vi "Add Points to Series_DBL-DBL[].vi"(6 "YValuesPerPoint":i32=1, 8 "error in (no error)":errorcluster, 9 "Data":cluster{"X":dbl, "Y":dbl[]}[](array[cluster])=[{"X"=0.0, "Y"=[]}, {"X"=0.0, "Y"=[]}, {"X"=0.0, "Y"=[]}, {"X"=0.0, "Y"=[]}, {"X"=0.0, "Y"=[]}, {"X"=0.0, "Y"=[]}, {"X"=0.0, "Y"=[]}, {"X"=0.0, "Y"=[]}], 10 ".NET MSChart Series":refnum<k24>) -> (0 "error out":errorcluster, 2 ".NET MSChart Series (dup)":refnum<k24>)   [LabVIEW 2014, in "XMSChart.xctl"]
uses:
  XMSChart.xctl
  System.Windows.Forms.DataVisualization
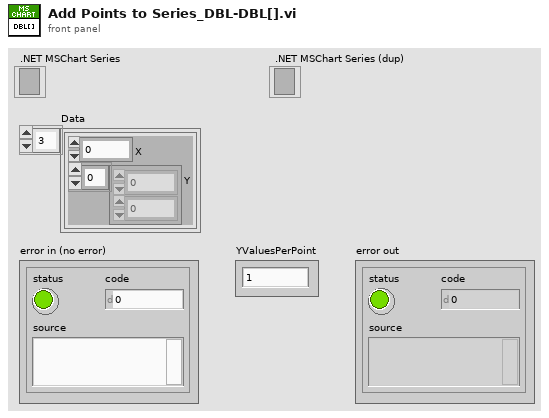
[diagram p1: front panel]
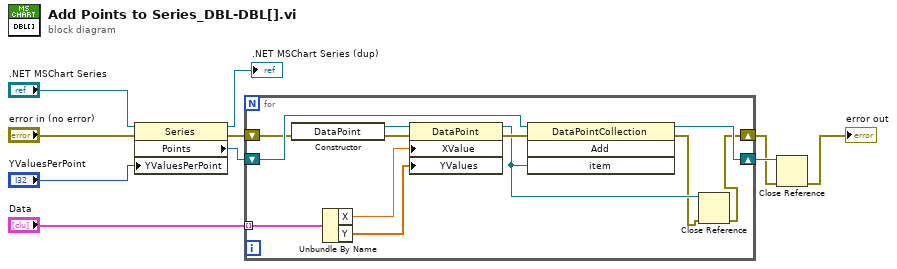
[diagram p0: block diagram]
diagram:
  n1 = property class="Series"(reference=".NET MSChart Series", error in="error in (no error)", "YValuesPerPoint"="YValuesPerPoint") -> (reference out=→".NET MSChart Series (dup)":refnum<k24>, error out=w6:errorcluster, "Points"=w7:refnum<k24>)
  n2 = for {
    shift-right: [w21] -> w4
    shift-left: w7 -> [w22]
    shift-right: [w11] -> w3
    shift-left: w6 -> [w17]
    tunnel: "Data" -> [w19] mode=indexing
    n3 = constructor class="DataPoint"(error in=w17) -> (reference out=w20:refnum<k24>, error out=w18:errorcluster)  [unwired: 2 in, 1 out]
    n4 = Unbundle By Name(w19) -> ("X"=w15:dbl, "Y"=w14:dbl[])
    n5 = property class="DataPoint"(reference=w20, error in=w18, "XValue"=w15, "YValues"=w14) -> (reference out=w13:refnum<k24>, error out=w16:errorcluster)
    n6 = invoke class="DataPointCollection" method="Add"(reference=w22, error in=w16, "item"=w13) -> (reference out=w21:refnum<k24>, error out=w12:errorcluster)  [unwired: 1 in, 2 out]
    n7 = Close Reference(reference=w13, error in (no error)=w12) -> (error out=w11:errorcluster)
  }
  n8 = Close Reference(reference=w4, error in (no error)=w3) -> (error out=→"error out":errorcluster)
